vi "svx_Polar_Execute.vi"(0 "Container State":T6, 1 "Polar Plot":refnum<vi>, 2 "Plot Legend":refnum<vi>, 3 "z scale graph":refnum<vi>, 4 "Cursor Info":refnum<vi>, 5 "Facade VI":refnum<vi>, 6 "current state":T1={"Property Name"=[], "Container bounds"={"Width"=550, "Height"=250}, "Scale range"={"Maximum"=1.0, "Increment"=1.0}, "PointIdx"=0, "Marker list"=[], "Color settings"={"Arrow color"=16860, "Magnitude major grid"=13816530, "Magnitude minor grid"=16777216, "Phase grid"=13816530, "Phase scale marker text"=0}, "Magnitude scale name"="Magnitude", "Magnitude scale format string"="%#.2e", "MagnitudeScale:Visible"=TRUE, "MagnitudeScaleLabel:Visible"=TRUE, "PhaseScale:Visible"=TRUE, "Marker:Visible"=TRUE, "Cursor:Visible"=FALSE, "CursorName:Visible"=TRUE, "Autoscale"=TRUE, "Marker color"=16860, "Line color"=16711680, "Cursor color"=16711680, "Magnitude scale marker color"=0, "Plot.Line Style"=0, "Plot.Line Width"=0, "Plot.Point Style"=0, "Cursor.Line Style"=0, "Cursor.Line Width"=0, "Cursor.Point Style"=0, "Cursor.Style"=4, "Marker.Point Style"=2, "Point/fill color"=16711680, "Background color"=16777225, "Cursor name"="", "Cursor Release"=refnum, "Scale Range Change"=refnum, "data size(s)"=[], "Selectors:Visible"=TRUE, "Selector:ring Strings"={"Selector:Custom Strings"=FALSE, "Selector:Row Strings []"=[], "Selector:Column Strings []"=[], "User:Row Strings []"=[], "User:Column Strings []"=[]}, "Lock Cursor Info Position"=FALSE, "CursLoc"={"magnitude"=0.0, "phase"=0.0, "time/rev/RPM"=0.0}, "Plot Area:Position"={"Left"=0, "Top"=0}, "Plot Area:Size"={"Width"=0, "Height"=0}, "Marker.Style"=0, "Indication Arcs"=[], "Arc.Selector"=0, "customized marker"=[], "tree Width"=0, " Parents Tags"=[], "Children Tags"=[], "open?"=[], "index"=[{"row index"=0, "column index"=0}], "Label"="", "custom strings changed"=FALSE, "Owning VI"=refnum, "Legend BG color"=16777225, "Legend font color"=0, "column Width"=203, "attribute"=variant} caption="State", 7 "To Do":T5[](array[typedef]), 8 "Data In":T4) -> (10 "Data Out":T4, 12 "Display State Out":T1={"Property Name"=[], "Container bounds"={"Width"=550, "Height"=250}, "Scale range"={"Maximum"=1.0, "Increment"=1.0}, "PointIdx"=0, "Marker list"=[], "Color settings"={"Arrow color"=16860, "Magnitude major grid"=13816530, "Magnitude minor grid"=16777216, "Phase grid"=13816530, "Phase scale marker text"=0}, "Magnitude scale name"="Magnitude", "Magnitude scale format string"="%#.2e", "MagnitudeScale:Visible"=TRUE, "MagnitudeScaleLabel:Visible"=TRUE, "PhaseScale:Visible"=TRUE, "Marker:Visible"=TRUE, "Cursor:Visible"=FALSE, "CursorName:Visible"=TRUE, "Autoscale"=TRUE, "Marker color"=16860, "Line color"=16711680, "Cursor color"=16711680, "Magnitude scale marker color"=0, "Plot.Line Style"=0, "Plot.Line Width"=0, "Plot.Point Style"=0, "Cursor.Line Style"=0, "Cursor.Line Width"=0, "Cursor.Point Style"=0, "Cursor.Style"=4, "Marker.Point Style"=2, "Point/fill color"=16711680, "Background color"=16777225, "Cursor name"="", "Cursor Release"=refnum, "Scale Range Change"=refnum, "data size(s)"=[], "Selectors:Visible"=TRUE, "Selector:ring Strings"={"Selector:Custom Strings"=FALSE, "Selector:Row Strings []"=[], "Selector:Column Strings []"=[], "User:Row Strings []"=[], "User:Column Strings []"=[]}, "Lock Cursor Info Position"=FALSE, "CursLoc"={"magnitude"=0.0, "phase"=0.0, "time/rev/RPM"=0.0}, "Plot Area:Position"={"Left"=0, "Top"=0}, "Plot Area:Size"={"Width"=0, "Height"=0}, "Marker.Style"=0, "Indication Arcs"=[], "Arc.Selector"=0, "customized marker"=[], "tree Width"=203, " Parents Tags"=[], "Children Tags"=[], "open?"=[], "index"=[{"row index"=0, "column index"=0}], "Label"="", "custom strings changed"=FALSE, "Owning VI"=refnum, "Legend BG color"=16777225, "Legend font color"=0, "column Width"=203, "attribute"=variant} caption="State")   [LabVIEW 2017, in "SVX Polar Plot.xctl"]
uses:
  <vilib>/addons/_XControls/Polar Plot/SVX Polar Plot.xctl
  <vilib>/addons/_XControls/Polar Plot/subVIs/svx_Polar_Plot_Data.ctl
  <vilib>/_xctls/Container State.ctl
  <vilib>/addons/_XControls/Polar Plot/subVIs/svx_Polar_Exe_Tasks.ctl
  <vilib>/addons/_XControls/Polar Plot/subVIs/svx_Polar_Plot_Internal_State.ctl
  <vilib>/addons/_XControls/Polar Plot/subVIs/svx_Polar_Indication_Arcs.ctl
  <vilib>/addons/_XControls/Polar Plot/subVIs/svx_Polar_Customized_Markers.ctl
  <vilib>/Utility/miscctls.llb/LVPointTypeDef.ctl
  <vilib>/Utility/miscctls.llb/LVAnnotationListTypeDef.ctl
  <vilib>/Utility/miscctls.llb/LVBoundsTypeDef.ctl
  <vilib>/_xctls/XControlSupport.lvlib
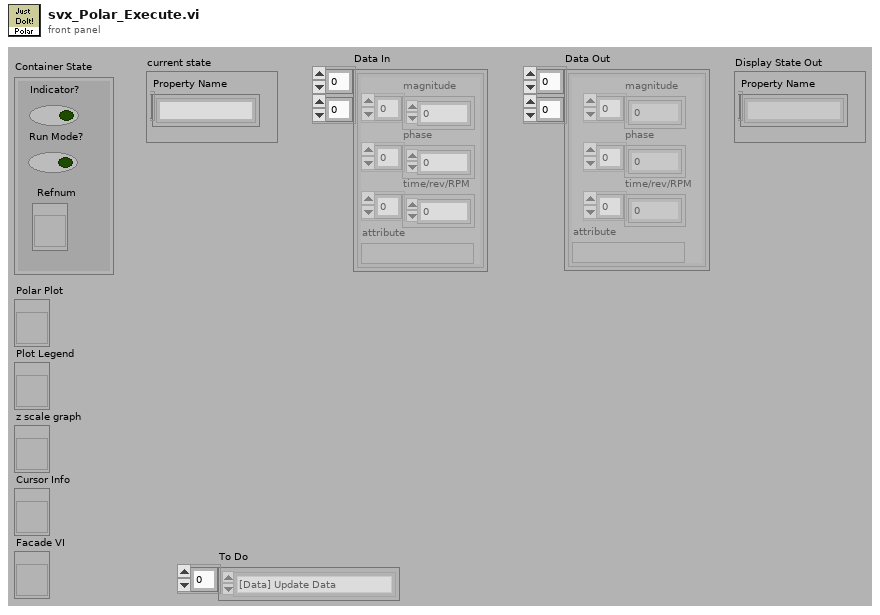
[diagram p1: front panel]
types:
  T1 = typedef "SVX Polar Plot.xctl/svx_Polar_Plot_Internal_State.ctl" = cluster{"Property Name":string[], "Container bounds":cluster{"Width":u32, "Height":u32}, "Scale range":cluster{"Maximum":dbl, "Increment":dbl}, "PointIdx":i32, "Marker list":cluster{"Name":string, "Color":u32, "Style":u8, "Point Style":u8, "Name Visible":bool, "Allow Drag":bool, "Annotation Mode":u32, "Plot":i32, "Index":i32, "Position":cluster{"X":dbl, "Y":dbl}, "X Scale":u32, "Y Scale":u32, "Show Arrow":bool, "Lock Name":bool, "Plot Area":i32, "Label Offset":cluster{"X":dbl, "Y":dbl}}[], "Color settings":cluster{"Arrow color":u32, "Magnitude major grid":u32, "Magnitude minor grid":u32, "Phase grid":u32, "Phase scale marker text":u32}, "Magnitude scale name":string, "Magnitude scale format string":string, "MagnitudeScale:Visible":bool, "MagnitudeScaleLabel:Visible":bool, "PhaseScale:Visible":bool, "Marker:Visible":bool, "Cursor:Visible":bool, "CursorName:Visible":bool, "Autoscale":bool, "Marker color":u32, "Line color":u32, "Cursor color":u32, "Magnitude scale marker color":u32, "Plot.Line Style":i32, "Plot.Line Width":i32, "Plot.Point Style":i32, "Cursor.Line Style":i32, "Cursor.Line Width":i32, "Cursor.Point Style":i32, "Cursor.Style":i32, "Marker.Point Style":i32, "Point/fill color":u32, "Background color":u32, "Cursor name":string, "Cursor Release":refnum<user-event>, "Scale Range Change":refnum<user-event>, "data size(s)":i32[], "Selectors:Visible":bool, "Selector:ring Strings":cluster{"Selector:Custom Strings":bool, "Selector:Row Strings []":string[], "Selector:Column Strings []":string[], "User:Row Strings []":string[], "User:Column Strings []":string[]}, "Lock Cursor Info Position":bool, "CursLoc":cluster{"magnitude":dbl, "phase":dbl, "time/rev/RPM":dbl}, "Plot Area:Position":cluster{"Left":i32, "Top":i32}, "Plot Area:Size":cluster{"Width":u32, "Height":u32}, "Marker.Style":i32, "Indication Arcs":T2, "Arc.Selector":u16, "customized marker":T3, "tree Width":u32, " Parents Tags":string[], "Children Tags":string[], "open?":bool[], "index":cluster{"row index":i32, "column index":i32}[], "Label":string, "custom strings changed":bool, "Owning VI":refnum<vi>, "Legend BG color":u32, "Legend font color":u32, "column Width":u32, "attribute":variant}
  T2 = typedef "SVX Polar Plot.xctl/svx_Polar_Indication_Arcs.ctl" = cluster{"Name":string, "Start radius":dbl, "End radius":dbl, "Line Style":i32, "Line Width":i32, "Border color":u32, "Fill color":u32, "Start angle":i16, "End angle":i16, "Visible":bool}[]
  T3 = typedef "SVX Polar Plot.xctl/svx_Polar_Customized_Markers.ctl" = cluster{"Name":string, "Color":u32, "Style":u8, "Point Style":u8, "Name Visible":bool, "Allow Drag":bool, "Annotation Mode":u32, "Plot":i32, "Index":i32, "Position":cluster{"Magnitude":dbl, "Phase":dbl}, "X Scale":u32, "Y Scale":u32, "Show Arrow":bool, "Lock Name":bool, "Plot Area":i32, "Label Offset":cluster{"Magnitude":dbl, "Phase":dbl}}[]
  T4 = typedef "SVX Polar Plot.xctl/svx_Polar_Plot_Data.ctl" = cluster{"magnitude":dbl[], "phase":dbl[], "time/rev/RPM":dbl[], "attribute":variant}[][]
  T5 = typedef "SVX Polar Plot.xctl/svx_Polar_Exe_Tasks.ctl" = enum16{"[Data] Update Data", "[Scale] Update Polar Scale", "[Scale] Autoscale", "[Legend] Update Legend", "[Cursor] Cursor Release", "[Pane] Change Minimum Size", "[Annt] Upodate Annotation", "[Plot] Appearance", "[Cursor] Visibility", "[Cursor] Appearance", "[Cursor] Index", "[Scale] MagnitudeVisibility", "[Scale] PhaseVisibility", "[Scale] PhaseAppearance", "[Scale] MagnitudeApperance", "[Plot] AcceptanceRegion", "[Scale] RangeChange", "[Marker] Appearance", "[Marker] List", "[Marker] Visibility", "[Legend] Visibility", "[Legend] Color", "[Data] Index", "[Legend] Update String", "[Cursor] Trigger Event", "[Scale] Trigger Event", "[Data] Clear Graph"}
  T6 = typedef "XControlSupport.lvlib/Container State.ctl" = cluster{"Indicator?":bool, "Run Mode?":bool, " Refnum":refnum<vi>}
  T7 = typedef "LVPointTypeDef.ctl" = cluster{"Horizontal":i16, "Vertical":i16}
  T8 = cluster{"Name":string, "Color":u32, "Style":u8, "Point Style":u8, "Name Visible":bool, "Allow Drag":bool, "Annotation Mode":u32, "Plot":i32, "Index":i32, "Position":cluster{"X":dbl, "Y":dbl}, "X Scale":u32, "Y Scale":u32, "Show Arrow":bool, "Lock Name":bool, "Plot Area":i32, "Label Offset":cluster{"X":dbl, "Y":dbl}}[]
  T9 = typedef "LVAnnotationListTypeDef.ctl" = cluster{"Name":string, "Color":u32, "Style":u8, "Point Style":u8, "Name Visible":bool, "Allow Drag":bool, "Annotation Mode":u32, "Plot":i32, "Index":i32, "Position":cluster{"X":dbl, "Y":dbl}, "X Scale":u32, "Y Scale":u32, "Show Arrow":bool, "Lock Name":bool, "Plot Area":i32, "Label Offset":cluster{"X":dbl, "Y":dbl}}[]
  T10 = typedef "LVBoundsTypeDef.ctl" = cluster{"Width":u32, "Height":u32}
  T11 = cluster{"PointIdx":i32, "Position":cluster{"Magnitude":dbl, "Phase":dbl, "Reference":dbl}}
  T12 = cluster{"Selector:Custom Strings":bool, "Selector:Row Strings []":string[], "Selector:Column Strings []":string[], "User:Row Strings []":string[], "User:Column Strings []":string[]}
  T13 = cluster{"magnitude":dbl[], "phase":dbl[], "time/rev/RPM":dbl[], "attribute":variant}
  T14 = cluster{"Arrow color":u32, "Magnitude major grid":u32, "Magnitude minor grid":u32, "Phase grid":u32, "Phase scale marker text":u32}
  T15 = cluster{"Numeric":dbl, "Numeric":dbl, "Numeric":dbl}
  T16 = typedef "LVCursorListTypeDef.ctl" = cluster{"Name":string, "Color":u32, "Style":u8, "Point Style":u8, "Name Visible":bool, "Allow Drag":bool, "Cursor Mode":u32, "Plot":i32, "Index":i32, "Position":cluster{"X":dbl, "Y":dbl}, "X Scale":u32, "Y Scale":u32, "Watch Plots":i32[], "Watch All Plots":bool, "Plot Area":i32, "Label Offset":cluster{"X":dbl, "Y":dbl}}[]
  T17 = cluster{"Name":string, "Color":u32, "Style":u8, "Point Style":u8, "Name Visible":bool, "Allow Drag":bool, "Cursor Mode":u32, "Plot":i32, "Index":i32, "Position":cluster{"X":dbl, "Y":dbl}, "X Scale":u32, "Y Scale":u32, "Watch Plots":i32[], "Watch All Plots":bool, "Plot Area":i32, "Label Offset":cluster{"X":dbl, "Y":dbl}}
  T18 = cluster{"Name":string, "Color":u32, "Style":u8, "Point Style":u8, "Name Visible":bool, "Allow Drag":bool, "Annotation Mode":u32, "Plot":i32, "Index":i32, "Position":cluster{"X":dbl, "Y":dbl}, "X Scale":u32, "Y Scale":u32, "Show Arrow":bool, "Lock Name":bool, "Plot Area":i32, "Label Offset":cluster{"X":dbl, "Y":dbl}}
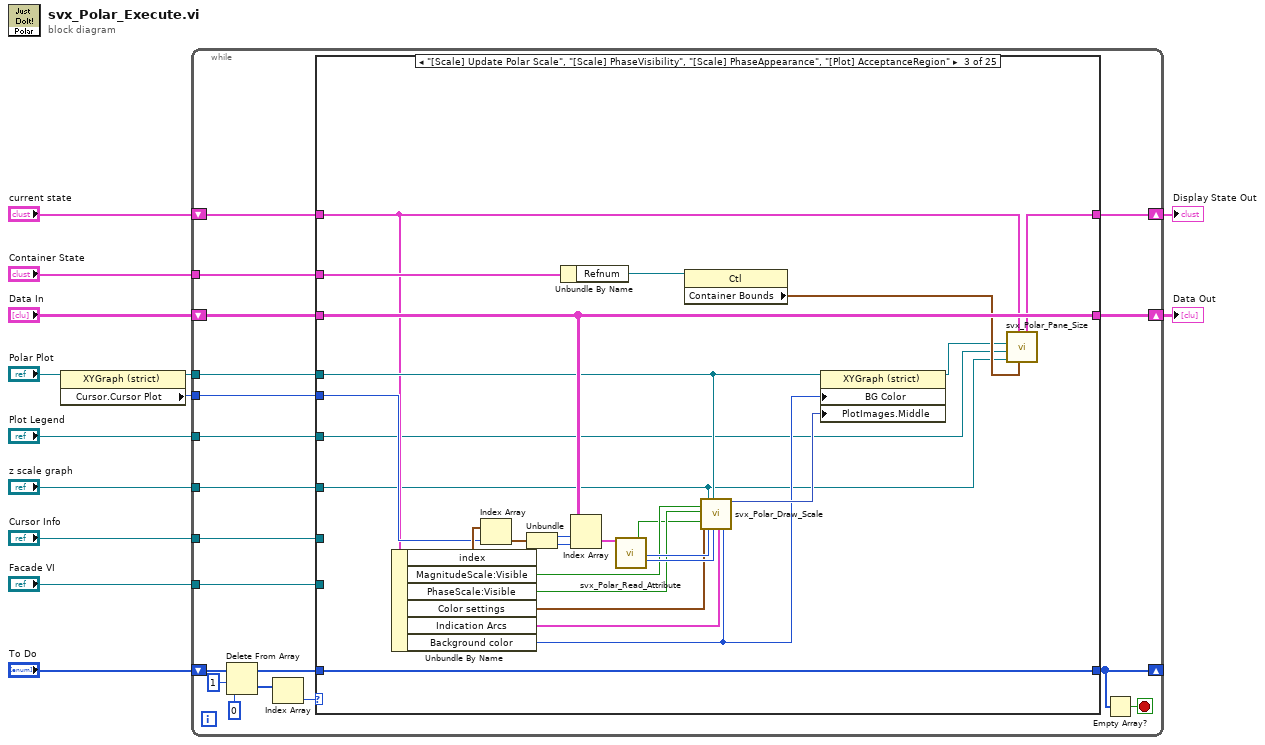
[diagram p0: block diagram]
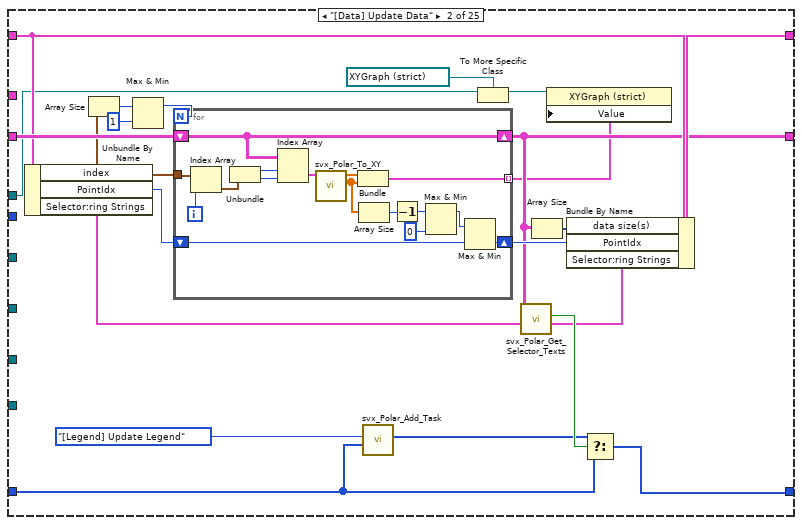
[diagram p3: hidden frame]
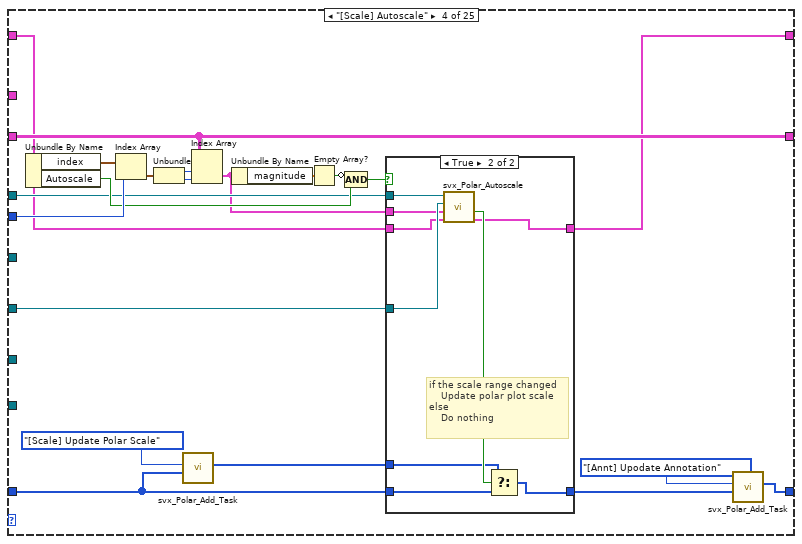
[diagram p4: hidden frame]
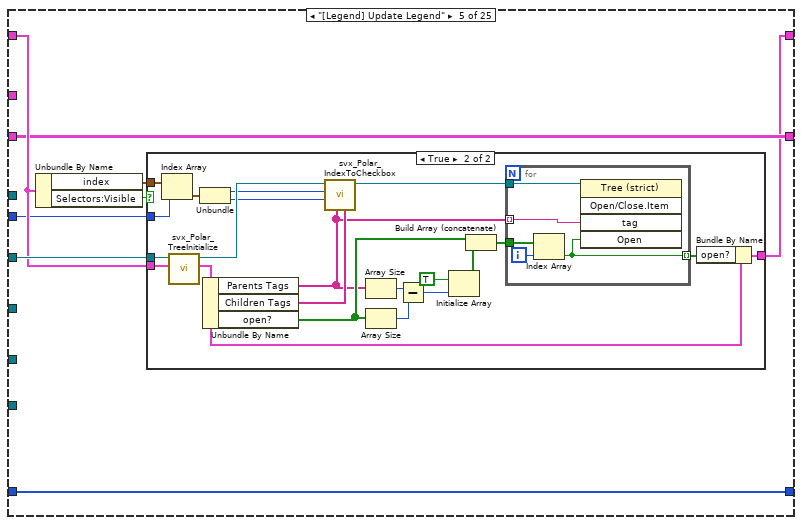
[diagram p6: hidden frame]
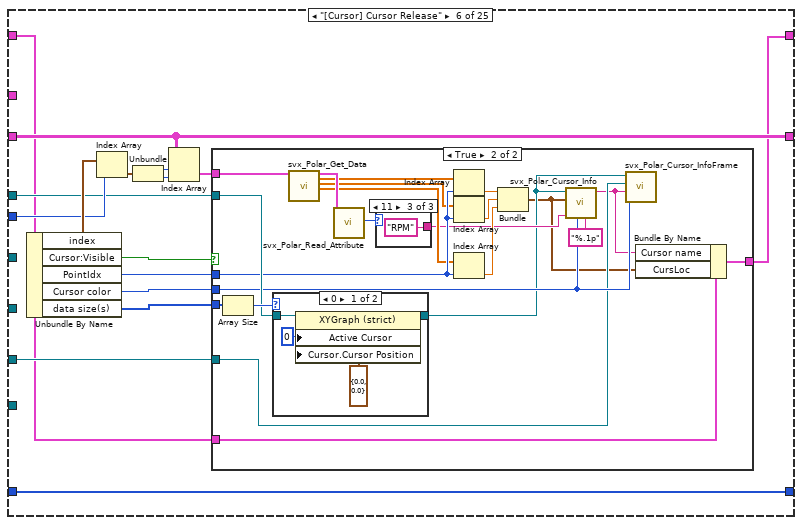
[diagram p8: hidden frame]
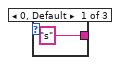
[diagram p10: hidden frame]
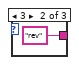
[diagram p11: hidden frame]
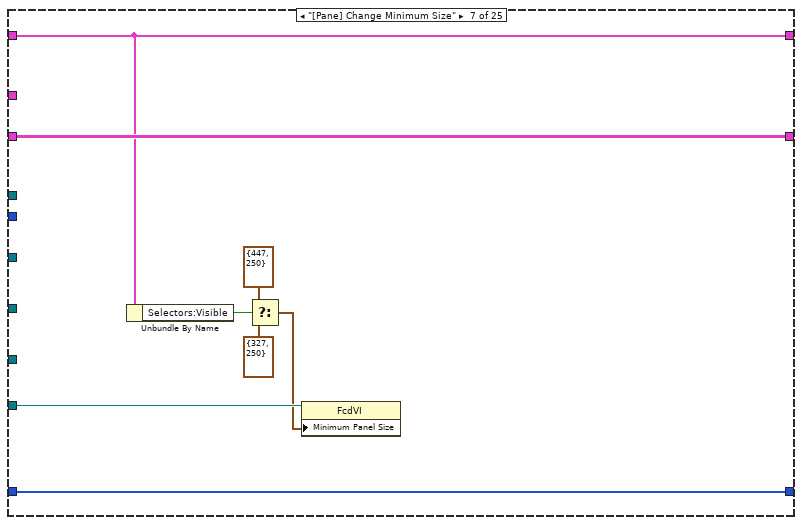
[diagram p13: hidden frame]
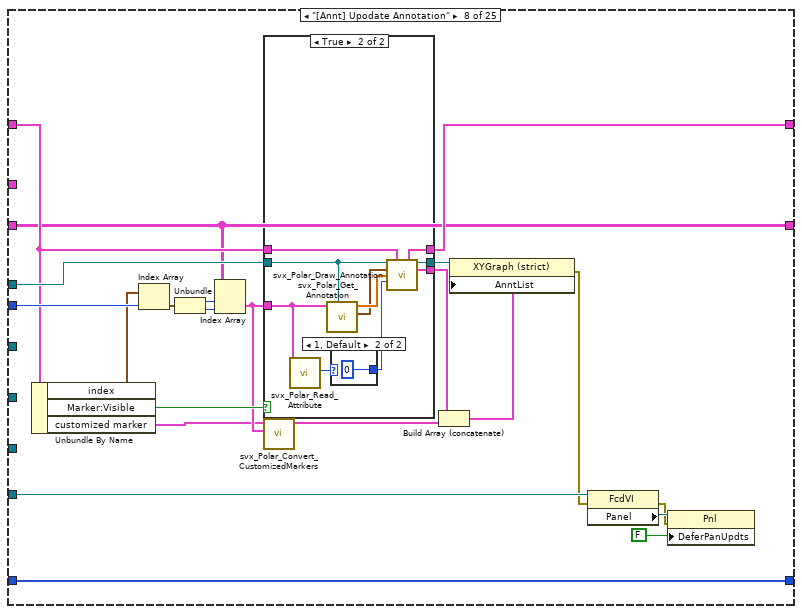
[diagram p14: hidden frame]
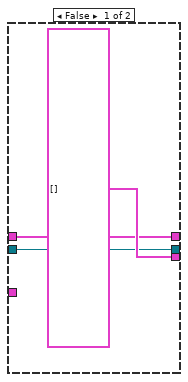
[diagram p15: hidden frame]
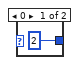
[diagram p16: hidden frame]
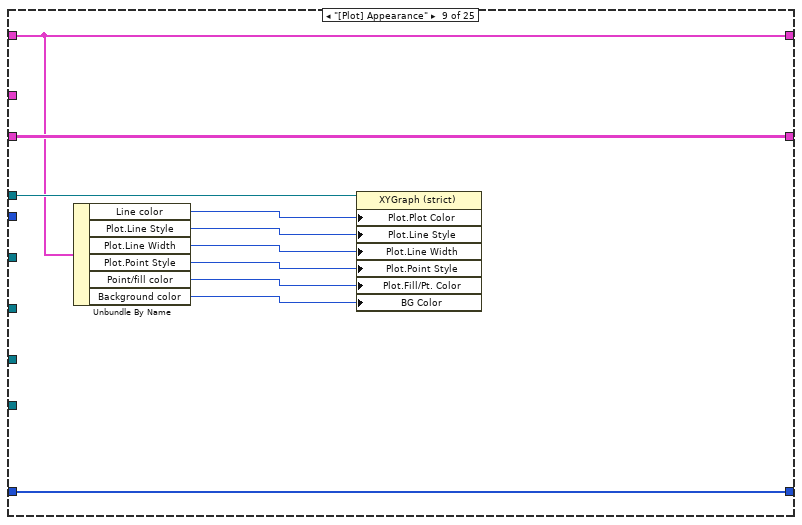
[diagram p17: hidden frame]
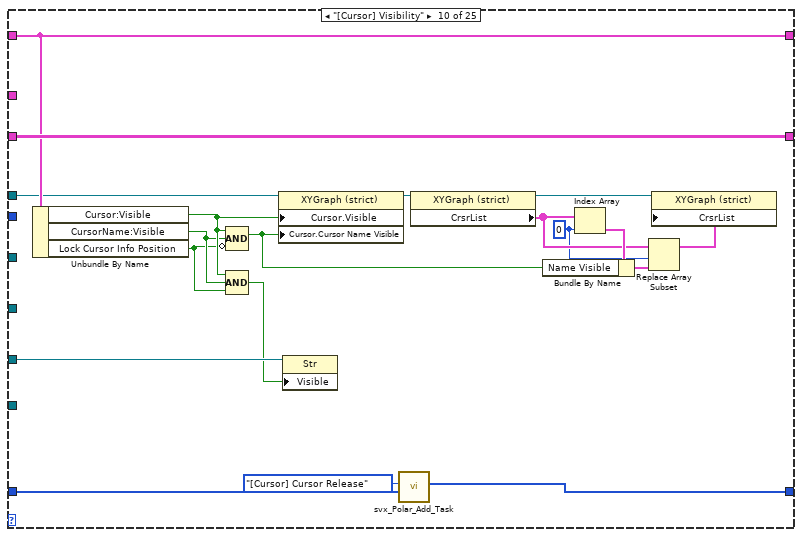
[diagram p18: hidden frame]
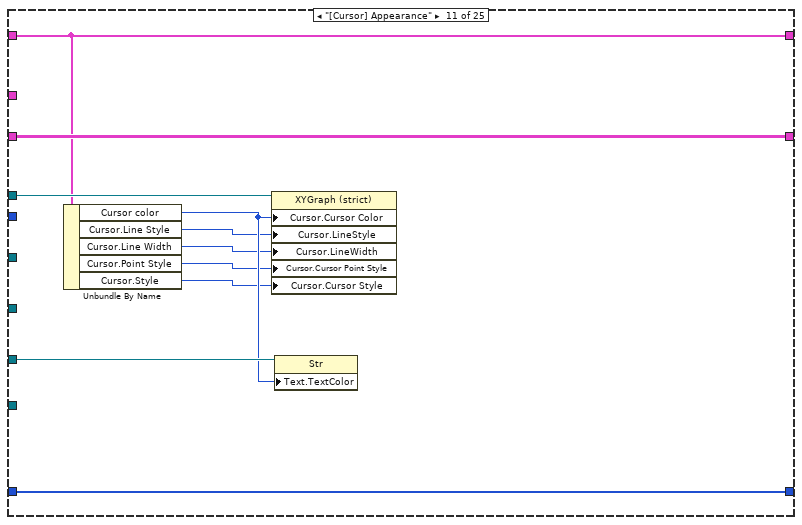
[diagram p19: hidden frame]
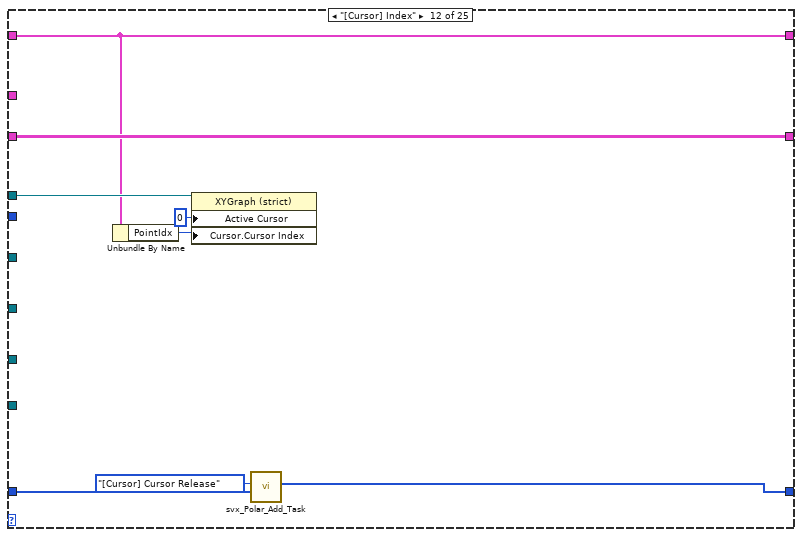
[diagram p20: hidden frame]
diagram:
  n1 = property class="XYGraph (strict)"(reference="Polar Plot") -> (reference out=w10:refnum<vi>, "Cursor.Cursor Plot"=w11:i32)  [unwired: 1 in, 1 out]
  n2 = while {
    shift-right: [w30] -> w6
    shift-left: "current state" -> [w32]
    shift-right: [w14] -> w5
    shift-left: "Data In" -> [w31]
    tunnel: w11 -> [w29]
    tunnel: w10 -> [w28]
    tunnel: "Plot Legend" -> [w27]
    tunnel: "z scale graph" -> [w26]
    tunnel: "Cursor Info" -> [w25]
    shift-right: [w15] -> _
    shift-left: "To Do" -> [w24]
    tunnel: "Facade VI" -> [w17]
    tunnel: "Container State" -> [w16]
    stop <- w19 stop-if-true
    n3 = Delete From Array(array=w24, length=1, index=0) -> (deleted portion=w21:T5[], array with subset deleted=w18:T5[])
    n4 = Index Array(array=w21) -> (element=w20:T5)  [unwired: 1 in]
    n5 = case shown="\"[Scale] Update Polar Scale\", \"[Scale] PhaseVisibility\", \"[Scale] PhaseAppearance\", \"[Plot] AcceptanceRegion\"" w20 {
      tunnel: w32 -> [w35 w55 w78 w107 w138 w169 w217 w236 w265 w283 w294 w301 w307 w329 w348 w363 w375 w392 w439 w447 w457 w469 w478 w484 w491]
      tunnel: w31 -> [w34 w57 w97 w117 w134 w177 w221 w226 w268 w284 w297 w305 w319 w342 w358 w365 w376 w384 w445 w452 w456 w462 w481 w486 _]
      tunnel: [w35 w53 w77 w106 w133 w168 w217 w235 w265 w283 w294 w301 w306 w328 w348 w361 w375 w393 w438 w447 w457 w470 w478 w484 w490] -> w30
      tunnel: w29 -> [_ _ w98 w118 w137 w178 _ w240 _ _ _ _ _ _ _ _ _ w386 _ _ _ _ _ _ _]
      tunnel: w28 -> [_ w43 w85 w110 _ w171 _ w237 w266 w282 w295 w302 w318 w330 w349 w362 w378 w391 w444 _ _ _ _ _ _]
      tunnel: w27 -> [_ _ w75 _ w139 _ _ _ _ _ _ _ w311 w327 _ _ _ _ w443 w446 _ _ _ _ _]
      tunnel: w26 -> [_ _ w74 w109 _ _ _ _ _ _ _ _ w317 w341 w350 _ _ _ w442 _ _ _ _ _ _]
      tunnel: w25 -> [_ _ _ _ _ w170 _ _ _ w278 w293 _ _ _ _ _ _ _ _ _ _ _ _ _ _]
      tunnel: w18 -> [w33 w45 w83 w103 w132 w167 w214 w227 w267 w287 w296 w300 w320 w336 w347 w364 w377 w396 w437 w451 w454 w464 w480 w485 w488]
      tunnel: [w33 w48 w83 w100 w132 w167 w214 w227 w267 w286 w296 w298 w320 w334 w343 w364 w377 w396 w436 w451 w453 w463 w480 w485 w487] -> w15
      tunnel: w17 -> [_ _ _ _ _ _ w216 w231 _ _ _ _ _ _ _ _ _ w383 _ _ _ _ _ _ _]
      tunnel: w16 -> [_ _ w79 _ _ _ _ _ _ _ _ _ w310 w331 _ _ _ _ w441 _ _ _ _ _ _]
      tunnel: [w34 w51 w97 w117 w134 w177 w221 w226 w268 w284 w297 w305 w319 w342 w358 w365 w376 w384 w445 w452 w456 w462 w481 w486 T4 [] ("Data In")] -> w14
      frame Default {
      }
      frame "[Data] Update Data" {
        n6 = Unbundle By Name(w55) -> ("index"=w36:cluster{"row index":i32, "column index":i32}[], "PointIdx"=w56:i32, "Selector:ring Strings"=w50:T12)
        n7 = Array Size(array=w36) -> (size(s)=w38:i32)
        n8 = Max & Min(x=w38, y=1 ("x")) -> (max(x,y)=w39:i32)  [unwired: 1 out]
        n9 = for {
          N: w39 -> [_]
          shift-right: [w73] -> w51
          shift-left: w57 -> [w73]
          tunnel: [w68] -> w40 mode=indexing
          shift-right: [w61] -> w54
          shift-left: w56 -> [w62]
          tunnel: w36 -> [w60]
          i -> [w59]
          n10 = Index Array(array=w60, index=w59) -> (element=w58:cluster{"row index":i32, "column index":i32})
          n11 = Unbundle(w58) -> ("row index"=w72:i32, "column index"=w71:i32)
          n12 = Index Array(array=w73, index (row)=w72, index (col)=w71) -> (element=w70:T13)
          n13 = call <vilib>:"svx_Polar_To_XY.vi"("polar plot"=w70) -> ("y"=w67:dbl[], "x"=w69:dbl[])  [unwired: 7 in, 2 out]
          n14 = Bundle("x"=w69, "y"=w67) -> (w68:cluster{"x":dbl[], "y":dbl[]})  [unwired: 1 in]
          n15 = Array Size(array=w67) -> (size(s)=w65:i32)
          n16 = Decrement(x=w65) -> (x-1=w66:i32)
          n17 = Max & Min(x=w66, y=0) -> (max(x,y)=w63:i32)  [unwired: 1 out]
          n18 = Max & Min(x=w63, y=w62) -> (min(x,y)=w61:i32)  [unwired: 1 out]
        }
        n19 = call <vilib>:"svx_Polar_Add_Task.vi"("task list"=w45, "new task"=svx_Polar_Exe_Tasks."[Legend] Update Legend" ("Tasks")) -> ("task list out"=w44:T5[])  [unwired: 9 in]
        n20 = To More Specific Class(target class=refnum<vi> refnum ("Polar Plot dummy"), reference=w43) -> (specific class reference=w41:refnum<vi>)  [unwired: 1 in, 1 out]
        n21 = call <vilib>:"svx_Polar_Get_Selector_Texts.vi"("Selector:ring Strings"=w50, "polar plot"=w51) -> ("Selector:ring Strings out"=w47:T12, "update legend?"=w49:bool)  [unwired: 7 in, 1 out]
        n22 = Array Size(array=w51) -> (size(s)=w52:i32[])
        n23 = property class="XYGraph (strict)"(reference=w41, "Value"=w40) -> ()  [unwired: 1 in, 2 out]
        n24 = Bundle By Name(cluster=w55, "data size(s)"=w52, "PointIdx"=w54, "Selector:ring Strings"=w47) -> (w53:T1)
        n25 = Select(t=w44, s=w49, f=w45) -> (s? t:f=w48:T5[])
      }
      frame "[Scale] Update Polar Scale", "[Scale] PhaseVisibility", "[Scale] PhaseAppearance", "[Plot] AcceptanceRegion" {
        n26 = Unbundle By Name(w78) -> ("index"=w99:cluster{"row index":i32, "column index":i32}[], "MagnitudeScale:Visible"=w89:bool, "PhaseScale:Visible"=w88:bool, "Color settings"=w86:T14, "Indication Arcs"=w90:T2, "Background color"=w82:u32)
        n27 = Index Array(array=w99, index=w98) -> (element=w96:cluster{"row index":i32, "column index":i32})
        n28 = Unbundle(w96) -> ("row index"=w95:i32, "column index"=w94:i32)
        n29 = Unbundle By Name(w79) -> ("Refnum"=w81:refnum<vi>)
        n30 = Index Array(array=w97, index (row)=w95, index (col)=w94) -> (element=w93:T13)
        n31 = call <vilib>:"svx_Polar_Read_Attribute.vi"("polar plot"=w93) -> ("is OA Polar Plot?"=w87:bool, "shaft rotating direction"=w92:u16, "probe angle [deg]"=w91:u16)  [unwired: 13 in, 3 out]
        n32 = property class="Ctl"(reference=w81) -> ("Container Bounds"=w80:T10)  [unwired: 1 in, 2 out]
        n33 = call <vilib>:"svx_Polar_Draw_Scale.vi"("horizontal line visible"=w89, "thetaScale visible"=w88, "draw rotating direct"=w87, "color settings"=w86, "z scale graph ref in"=w74, "shaft rotating direction"=w92, "Polar Plot ref in"=w85, "probe angle [deg]"=w91, "Indication Arcs"=w90, "Background color"=w82) -> ("new picture"=w84:picture)  [unwired: 9 in]
        n34 = property class="XYGraph (strict)"(reference=w85, "BG Color"=w82, "PlotImages.Middle"=w84) -> (reference out=w76:refnum<vi>)  [unwired: 1 in, 1 out]
        n35 = call <vilib>:"svx_Polar_Pane_Size.vi"("Container bounds"=w80, "Display State In"=w78, "z scale graph Refnum"=w74, "Plot Legend Refnum"=w75, "Polar Plot Refnum in"=w76) -> ("Display State out"=w77:T1)  [unwired: 3 in, 3 out]
      }
      frame "[Scale] Autoscale" {
        n36 = Unbundle By Name(w107) -> ("index"=w119:cluster{"row index":i32, "column index":i32}[], "Autoscale"=w112:bool)
        n37 = Index Array(array=w119, index=w118) -> (element=w120:cluster{"row index":i32, "column index":i32})
        n38 = Unbundle(w120) -> ("row index"=w116:i32, "column index"=w115:i32)
        n39 = call <vilib>:"svx_Polar_Add_Task.vi"("task list"=w103, "new task"=svx_Polar_Exe_Tasks."[Scale] Update Polar Scale" ("element")) -> ("task list out"=w102:T5[])  [unwired: 9 in]
        n40 = Index Array(array=w117, index (row)=w116, index (col)=w115) -> (element=w108:T13)
        n41 = Unbundle By Name(w108) -> ("magnitude"=w113:dbl[])
        n42 = Empty Array?(array=w113) -> (empty?=w114:bool)
        n43 = Compound Arithmetic op=AND(invert w114, w112) -> (w111:bool)
        n44 = case shown="True" w111 {
          tunnel: w110 -> [_ w131]
          tunnel: w109 -> [_ w130]
          tunnel: w108 -> [_ w129]
          tunnel: w107 -> [w121 w128]
          tunnel: w103 -> [w122 w125]
          tunnel: w102 -> [_ w126]
          tunnel: [w122 w124] -> w101
          tunnel: [w121 w123] -> w106
          frame False {
          }
          frame True {
            # "if the scale range changed\n    Update polar plot scale\nelse\n    Do nothing"
            n45 = call <vilib>:"svx_Polar_Autoscale.vi"("State"=w128, "polar plot"=w129, "z scale graph"=w130, "Polar Plot"=w131) -> ("State out"=w123:T1, "redraw scale?"=w127:bool)  [unwired: 4 in, 2 out]
            n46 = Select(t=w126, s=w127, f=w125) -> (s? t:f=w124:T5[])
          }
        }
        n47 = call <vilib>:"svx_Polar_Add_Task.vi"("task list"=w101, "new task"=svx_Polar_Exe_Tasks."[Annt] Upodate Annotation" ("element")) -> ("task list out"=w100:T5[])  [unwired: 9 in]
      }
      frame "[Legend] Update Legend" {
        n48 = Unbundle By Name(w138) -> ("index"=w135:cluster{"row index":i32, "column index":i32}[], "Selectors:Visible"=w136:bool)
        n49 = case shown="True" w136 {
          tunnel: w139 -> [_ w161]
          tunnel: w138 -> [w140 w160]
          tunnel: w135 -> [_ w157]
          tunnel: w137 -> [_ w156]
          tunnel: [w140 w141] -> w133
          frame False {
          }
          frame True {
            n50 = Index Array(array=w157, index=w156) -> (element=w158:cluster{"row index":i32, "column index":i32})
            n51 = call <vilib>:"svx_Polar_TreeInitialize.vi"("Display State In"=w160, "Tree ref in"=w161) -> ("Display State out"=w143:T1, "Tree ref out"=w159:refnum<vi>)  [unwired: 6 in, 2 out]
            n52 = Unbundle(w158) -> ("row index"=w154:i32, "column index"=w155:i32)
            n53 = Unbundle By Name(w143) -> ("Parents Tags"=w146:string[], "Children Tags"=w153:string[], "open?"=w147:bool[])
            n54 = call <vilib>:"svx_Polar_IndexToCheckbox.vi"("All Children Tags"=w153, "All parents Tags"=w146, "ColumnIdx"=w155, "RowIdx"=w154, "Tree ref in"=w159) -> ("Tree ref out"=w144:refnum<vi>)  [unwired: 6 in]
            n55 = Array Size(array=w146) -> (size(s)=w150:i32)
            n56 = Array Size(array=w147) -> (size(s)=w149:i32)
            n57 = Subtract(x=w150, y=w149) -> (x-y=w151:i32)
            n58 = Initialize Array(TRUE, w151) -> (w148:bool[])
            n59 = Build Array (concatenate)(w147, w148) -> (w145:bool[])
            n60 = for {
              tunnel: w144 -> [w166]
              tunnel: w146 -> [w163] mode=indexing
              tunnel: w145 -> [w165]
              tunnel: [w162] -> w142 mode=indexing
              i -> [w164]
              n61 = Index Array(array=w165, index=w164) -> (element=w162:bool)
              n62 = invoke class="Tree (strict)" method="Open/Close.Item"(reference=w166, "tag"=w163, "Open"=w162) -> ()  [unwired: 2 in, 5 out]
            }
            n63 = Bundle By Name(cluster=w143, "open?"=w142) -> (w141:T1)
          }
        }
      }
      frame "[Cursor] Cursor Release" {
        n64 = Unbundle By Name(w169) -> ("index"=w182:cluster{"row index":i32, "column index":i32}[], "Cursor:Visible"=w175:bool, "PointIdx"=w174:i32, "Cursor color"=w173:u32, "data size(s)"=w172:i32[])
        n65 = Index Array(array=w182, index=w178) -> (element=w181:cluster{"row index":i32, "column index":i32})
        n66 = Unbundle(w181) -> ("row index"=w180:i32, "column index"=w179:i32)
        n67 = Index Array(array=w177, index (row)=w180, index (col)=w179) -> (element=w176:T13)
        n68 = case shown="True" w175 {
          tunnel: w176 -> [_ w188]
          tunnel: w174 -> [_ w197]
          tunnel: w173 -> [_ w191]
          tunnel: w172 -> [_ w204]
          tunnel: w171 -> [_ w203]
          tunnel: w170 -> [_ w189]
          tunnel: w169 -> [w183 w187]
          tunnel: [w183 w184] -> w168
          frame False {
          }
          frame True {
            n69 = Array Size(array=w204) -> (size(s)=w205:i32)
            n70 = case shown="0" w205 {
              tunnel: w203 -> [w210 w213]
              tunnel: [w209 w213] -> w190
              frame 0 {
                n71 = property on="Property Node" class="XYGraph (strict)"(reference=w210, "Active Cursor"=u32 0, "Cursor.Cursor Position"=cluster{"Cursor X":dbl, "Cursor Y":dbl} {"Cursor X"=0.0, "Cursor Y"=0.0}) -> (reference out=w209:refnum<vi>)  [unwired: 1 in, 1 out]
              }
              frame 1, Default {
              }
            }
            n72 = call <vilib>:"svx_Polar_Get_Data.vi"("polar plot"=w188) -> ("polar plot out"=w201:T13, "magnitude"=w196:dbl[], "phase"=w195:dbl[], "time/rev/RPM"=w194:dbl[])  [unwired: 13 in, 2 out]
            n73 = call <vilib>:"svx_Polar_Read_Attribute.vi"("polar plot"=w201) -> ("reference label"=w202:u16)  [unwired: 13 in, 5 out]
            n74 = case shown="11" w202 {
              tunnel: ["s" "rev" "RPM"] -> w192
              frame 0, Default {
              }
              frame 3 {
              }
              frame 11 {
              }
            }
            n75 = Index Array(array=w196, index=w197) -> (element=w198:dbl)
            n76 = Index Array(array=w195, index=w197) -> (element=w199:dbl)
            n77 = Index Array(array=w194, index=w197) -> (element=w200:dbl)
            n78 = Bundle("Numeric"=w198, "Numeric"=w199, "Numeric"=w200) -> (w185:T15)  [unwired: 1 in]
            n79 = call <vilib>:"svx_Polar_Cursor_Info.vi"("format string"="%.1p", "cursor color(blue)"=w191, "mark unit"=w192, "CursLoc"=w185, "Polar Plot"=w190) -> ("cursor name"=w186:string)  [unwired: 6 in]
            n80 = call <vilib>:"svx_Polar_Cursor_InfoFrame.vi"("Cursor color"=w191, "format string"=w186, "Cursor Info"=w189, "Polar Plot"=w190) -> ()  [unwired: 8 in]
            n81 = Bundle By Name(cluster=w187, "Cursor name"=w186, "CursLoc"=w185) -> (w184:T1)
          }
        }
      }
      frame "[Pane] Change Minimum Size" {
        n82 = Unbundle By Name(w217) -> ("Selectors:Visible"=w220:bool)
        n83 = Select(t=T7 {"Horizontal"=447, "Vertical"=250} ("Front Panel Window:Minimum Size"), s=w220, f=T7 {"Horizontal"=327, "Vertical"=250} ("Front Panel Window:Minimum Size")) -> (s? t:f=w215:T7)
        n84 = property class="FcdVI"(reference=w216, "Minimum Panel Size"=w215) -> ()  [unwired: 1 in, 2 out]
      }
      frame "[Annt] Upodate Annotation" {
        n85 = Unbundle By Name(w236) -> ("index"=w239:cluster{"row index":i32, "column index":i32}[], "Marker:Visible"=w238:bool, "customized marker"=w224:T3)
        n86 = Index Array(array=w239, index=w240) -> (element=w243:cluster{"row index":i32, "column index":i32})
        n87 = Unbundle(w243) -> ("row index"=w242:i32, "column index"=w241:i32)
        n88 = Index Array(array=w226, index (row)=w242, index (col)=w241) -> (element=w234:T13)
        n89 = case shown="True" w238 {
          tunnel: w234 -> [_ w252]
          tunnel: w237 -> [w244 w251]
          tunnel: w236 -> [w245 w250]
          tunnel: [w245 w249] -> w235
          tunnel: [T8 [] ("AnntList") w248] -> w233
          tunnel: [w244 w247] -> w232
          frame False {
          }
          frame True {
            n90 = call <vilib>:"svx_Polar_Read_Attribute.vi"("polar plot"=w252) -> ("reference label"=w256:u16)  [unwired: 13 in, 5 out]
            n91 = call <vilib>:"svx_Polar_Get_Annotation.vi"("Polar Plot"=w251, "data"=w252) -> ("Array"=w253:cluster{dbl, dbl}[], "marker value"=w254:dbl[])  [unwired: 8 in]
            n92 = case shown="1, Default" w256 {
              tunnel: [i16 2 ("precision (6)") i16 0 ("precision (6)")] -> w255
              frame 0 {
              }
              frame 1, Default {
              }
            }
            n93 = call <vilib>:"svx_Polar_Draw_Annotation.vi"("Polar Plot ref in"=w251, "State in"=w250, "position array"=w253, "Annotation Values"=w254, "precision (6)"=w255) -> ("State out"=w249:T1, "Polar Plot ref out"=w247:refnum<vi>, "AnntList"=w248:T9)  [unwired: 8 in]
          }
        }
        n94 = call <vilib>:"svx_Polar_Convert_CustomizedMarkers.vi"("polar plot"=w234, "customized marker"=w224) -> ("customized annotations"=w222:T9)  [unwired: 9 in]
        n95 = Build Array (concatenate)(w233, w222) -> (w223:T9)
        n96 = property class="XYGraph (strict)"(reference=w232, "AnntList"=w223) -> (error out=w230:errorcluster)  [unwired: 1 in, 1 out]
        n97 = property class="FcdVI"(reference=w231, error in=w230) -> (error out=w225:errorcluster, "Panel"=w229:refnum<vi>)  [unwired: 1 out]
        n98 = property class="Pnl"(reference=w229, error in=w225, "DeferPanUpdts"=FALSE ("Defer Panel Updates")) -> ()  [unwired: 2 out]
      }
      frame "[Plot] Appearance" {
        n99 = Unbundle By Name(w265) -> ("Line color"=w264:u32, "Plot.Line Style"=w263:i32, "Plot.Line Width"=w262:i32, "Plot.Point Style"=w261:i32, "Point/fill color"=w260:u32, "Background color"=w259:u32)
        n100 = property class="XYGraph (strict)"(reference=w266, "Plot.Plot Color"=w264, "Plot.Line Style"=w263, "Plot.Line Width"=w262, "Plot.Point Style"=w261, "Plot.Fill/Pt. Color"=w260, "BG Color"=w259) -> ()  [unwired: 1 in, 2 out]
      }
      frame "[Cursor] Visibility" {
        w274 = 0 ("index")
        n101 = Unbundle By Name(w283) -> ("Cursor:Visible"=w281:bool, "CursorName:Visible"=w280:bool, "Lock Cursor Info Position"=w279:bool)
        n102 = Compound Arithmetic op=AND(w281, w280, invert w279) -> (w271:bool)
        n103 = Compound Arithmetic op=AND(w281, w280, w279) -> (w277:bool)
        n104 = property class="XYGraph (strict)"(reference=w282, "Cursor.Visible"=w281, "Cursor.Cursor Name Visible"=w271) -> (reference out=w270:refnum<vi>)  [unwired: 1 in, 1 out]
        n105 = property class="Str"(reference=w278, "Visible"=w277) -> ()  [unwired: 1 in, 2 out]
        n106 = call <vilib>:"svx_Polar_Add_Task.vi"("task list"=w287, "new task"=svx_Polar_Exe_Tasks."[Cursor] Cursor Release") -> ("task list out"=w286:T5[])  [unwired: 9 in]
        n107 = property class="XYGraph (strict)"(reference=w270) -> (reference out=w272:refnum<vi>, "CrsrList"=w275:T16)  [unwired: 1 in, 1 out]
        n108 = Index Array(array=w275, index=w274) -> (element=w276:T17)
        n109 = Bundle By Name(cluster=w276, "Name Visible"=w271) -> (w273:T17)
        n110 = Replace Array Subset(array=w275, new element=w273, index=w274) -> (w269:T16)
        n111 = property class="XYGraph (strict)"(reference=w272, "CrsrList"=w269) -> ()  [unwired: 1 in, 2 out]
      }
      frame "[Cursor] Appearance" {
        n112 = Unbundle By Name(w294) -> ("Cursor color"=w292:u32, "Cursor.Line Style"=w291:i32, "Cursor.Line Width"=w290:i32, "Cursor.Point Style"=w289:i32, "Cursor.Style"=w288:i32)
        n113 = property class="XYGraph (strict)"(reference=w295, "Cursor.Cursor Color"=w292, "Cursor.LineStyle"=w291, "Cursor.LineWidth"=w290, "Cursor.Cursor Point Style"=w289, "Cursor.Cursor Style"=w288) -> ()  [unwired: 1 in, 2 out]
        n114 = property class="Str"(reference=w293, "Text.TextColor"=w292) -> ()  [unwired: 1 in, 2 out]
      }
      frame "[Cursor] Index" {
        n115 = Unbundle By Name(w301) -> ("PointIdx"=w304:i32)
        n116 = property class="XYGraph (strict)"(reference=w302, "Active Cursor"=u32 0, "Cursor.Cursor Index"=w304) -> ()  [unwired: 1 in, 2 out]
        n117 = call <vilib>:"svx_Polar_Add_Task.vi"("task list"=w300, "new task"=svx_Polar_Exe_Tasks."[Cursor] Cursor Release") -> ("task list out"=w298:T5[])  [unwired: 9 in]
      }
      frame "[Scale] MagnitudeVisibility" {
        n118 = Unbundle By Name(w307) -> ("MagnitudeScale:Visible"=w314:bool, "MagnitudeScaleLabel:Visible"=w315:bool)
        n119 = Unbundle By Name(w310) -> ("Refnum"=w309:refnum<vi>)
        n120 = property class="XYGraph (strict)"(reference=w317, "Visible"=w314, "YScale.NameLbl.Visible"=w315) -> (reference out=w316:refnum<vi>)  [unwired: 1 in, 1 out]
        n121 = property class="Ctl"(reference=w309) -> ("Container Bounds"=w308:T10)  [unwired: 1 in, 2 out]
        n122 = case shown="False" w314 {
          tunnel: w318 -> [w322 w325]
          tunnel: w316 -> [w321 w323]
          tunnel: [w322 w324] -> w313
          tunnel: [w321 w323] -> w312
          frame False {
          }
          frame True {
            n123 = call <vilib>:"svx_Polar_Align_Plot_Area.vi"("z scale graph ref in"=w323, "Polar Plot ref in"=w325) -> ("Polar Plot ref out"=w324:refnum<vi>)  [unwired: 8 in, 1 out]
          }
        }
        n124 = call <vilib>:"svx_Polar_Pane_Size.vi"("Container bounds"=w308, "Display State In"=w307, "z scale graph Refnum"=w312, "Plot Legend Refnum"=w311, "Polar Plot Refnum in"=w313) -> ("Display State out"=w306:T1)  [unwired: 3 in, 3 out]
      }
      frame "[Scale] MagnitudeApperance" {
        n125 = Unbundle By Name(w329) -> ("Color settings.Magnitude major grid"=w340:u32, "Magnitude scale marker color"=w339:u32, "Magnitude scale name"=w338:string, "Magnitude scale format string"=w337:string)
        n126 = Unbundle By Name(w331) -> ("Refnum"=w333:refnum<vi>)
        n127 = property class="Ctl"(reference=w333) -> ("Container Bounds"=w332:T10)  [unwired: 1 in, 2 out]
        n128 = property class="XYGraph (strict)"(reference=w341, "YScale.MinorTickColor"=w340, "YScale.TickColor"=w340, "YScale.Text Color"=w339, "YScale.NameLbl.Text"=w338, "YScale.FormatString"=w337) -> (reference out=w326:refnum<vi>)  [unwired: 1 in, 1 out]
        n129 = call <vilib>:"svx_Polar_Add_Task.vi"("task list"=w336, "new task"=svx_Polar_Exe_Tasks."[Scale] Update Polar Scale") -> ("task list out"=w334:T5[])  [unwired: 9 in]
        n130 = call <vilib>:"svx_Polar_Pane_Size.vi"("Container bounds"=w332, "Display State In"=w329, "z scale graph Refnum"=w326, "Plot Legend Refnum"=w327, "Polar Plot Refnum in"=w330) -> ("Display State out"=w328:T1)  [unwired: 3 in, 3 out]
      }
      frame "[Scale] RangeChange" {
        n131 = Unbundle By Name(w348) -> ("Scale range.Maximum"=w355:dbl)
        n132 = Negate(x=w355) -> (-x=w351:dbl)
        n133 = call <vilib>:"svx_Polar_Add_Task.vi"("task list"=w347, "new task"=svx_Polar_Exe_Tasks."[Scale] Update Polar Scale") -> ("task list out"=w345:T5[])  [unwired: 9 in]
        n134 = property on="Property Node" class="XYGraph (strict)"(reference=w349, "XScale.Maximum"=w355, "XScale.Minimum"=w351, "YScale.Maximum"=w355, "YScale.Minimum"=w351) -> (reference out=w356:refnum<vi>, error out=w354:errorcluster)  [unwired: 1 in]
        n135 = call <vilib>:"svx_Polar_Add_Task.vi"("task list"=w345, "new task"=svx_Polar_Exe_Tasks."[Annt] Upodate Annotation") -> ("task list out"=w343:T5[])  [unwired: 9 in]
        n136 = property on="Property Node" class="XYGraph (strict)"(reference=w350, error in=w354, "YScale.Flipped"=FALSE ("Y Scale.Flipped"), "YScale.Maximum"=w355, "YScale.Minimum"=0.0 ("Minimum")) -> (reference out=w357:refnum<vi>)  [unwired: 1 out]
        n137 = call <vilib>:"svx_Polar_Align_Plot_Area.vi"("z scale graph ref in"=w357, "Polar Plot ref in"=w356) -> ()  [unwired: 8 in, 2 out]
      }
      frame "[Marker] Appearance" {
        n138 = Unbundle By Name(w363) -> ("Marker color"=w369:u32, "Marker.Point Style"=w360:i32, "Marker.Style"=w359:i32)
        n139 = property class="XYGraph (strict)"(reference=w362) -> (reference out=w366:refnum<vi>, "AnntList"=w367:T9)  [unwired: 1 in, 1 out]
        n140 = for {
          tunnel: w367 -> [w374] mode=indexing
          tunnel: w369 -> [w373]
          tunnel: [w372] -> w368 mode=indexing
          tunnel: w360 -> [w371]
          tunnel: w359 -> [w370]
          n141 = Bundle By Name(cluster=w374, "Color"=w373, "Point Style"=w371, "Style"=w370) -> (w372:T18)
        }
        n142 = Bundle By Name(cluster=w363, "Marker list"=w368) -> (w361:T1)
        n143 = property class="XYGraph (strict)"(reference=w366, "AnntList"=w368) -> ()  [unwired: 1 in, 2 out]
      }
      frame "[Marker] List" {
        n144 = Unbundle By Name(w375) -> ("Marker list"=w379:T8)
        n145 = property on="Property Node" class="XYGraph (strict)"(reference=w378, "AnntList"=w379) -> (reference out=w380:refnum<vi>)  [unwired: 1 in, 1 out]
        n146 = property on="Property Node" class="XYGraph (strict)"(reference=w380) -> (reference out=w381:refnum<vi>, "AnntList"=w382:T9)  [unwired: 1 in, 1 out]
        n147 = property on="Property Node" class="XYGraph (strict)"(reference=w381, "AnntList"=w382) -> ()  [unwired: 1 in, 2 out]
      }
      frame "[Marker] Visibility" {
        n148 = Unbundle By Name(w392) -> ("Marker:Visible"=w394:bool, "customized marker"=w395:T3, "index"=w387:cluster{"row index":i32, "column index":i32}[])
        n149 = Index Array(array=w387, index=w386) -> (element=w390:cluster{"row index":i32, "column index":i32})
        n150 = Unbundle(w390) -> ("row index"=w389:i32, "column index"=w388:i32)
        n151 = Index Array(array=w384, index (row)=w389, index (col)=w388) -> (element=w385:T13)
        n152 = case shown="True" w394 {
          selector: w394 -> [w406 _]
          tunnel: w392 -> [w407 w419]
          tunnel: w391 -> [w399 w425]
          tunnel: w385 -> [w400 w415]
          tunnel: [w405 w420] -> w393
          tunnel: w395 -> [w398 w409]
          tunnel: w383 -> [_ w413]
          frame False {
            n153 = call <vilib>:"svx_Polar_Convert_CustomizedMarkers.vi"("polar plot"=w400, "customized marker"=w398) -> ("customized annotations"=w397:T9)  [unwired: 9 in]
            n154 = property class="XYGraph (strict)"(reference=w399, "AnntList"=w397) -> (reference out=w401:refnum<vi>)  [unwired: 1 in, 1 out]
            n155 = property class="XYGraph (strict)"(reference=w401) -> (reference out=w403:refnum<vi>, "AnntList"=w402:T9)  [unwired: 1 in, 1 out]
            n156 = Bundle By Name(cluster=w407, "Marker:Visible"=w406, "Marker list"=T9 [] ("Annotation List")) -> (w405:T1)
            n157 = property class="XYGraph (strict)"(reference=w403, "AnntList"=w402) -> ()  [unwired: 1 in, 2 out]
          }
          frame True {
            # "Do NOT remove this Read/Write operations.\nIt's not redundant. It is used to solve a update problem."
            n158 = call <vilib>:"svx_Polar_Read_Attribute.vi"("polar plot"=w415) -> ("reference label"=w418:u16)  [unwired: 13 in, 5 out]
            n159 = call <vilib>:"svx_Polar_Get_Annotation.vi"("Polar Plot"=w425, "data"=w415) -> ("Array"=w426:cluster{dbl, dbl}[], "marker value"=w427:dbl[])  [unwired: 8 in]
            n160 = case shown="1, Default" w418 {
              tunnel: [i16 2 ("precision (6)") i16 0 ("precision (6)")] -> w428
              frame 0 {
              }
              frame 1, Default {
              }
            }
            n161 = call <vilib>:"svx_Polar_Draw_Annotation.vi"("Polar Plot ref in"=w425, "State in"=w419, "position array"=w426, "Annotation Values"=w427, "precision (6)"=w428) -> ("State out"=w422:T1, "Polar Plot ref out"=w414:refnum<vi>, "AnntList"=w416:T9)  [unwired: 8 in]
            n162 = call <vilib>:"svx_Polar_Convert_CustomizedMarkers.vi"("polar plot"=w415, "customized marker"=w409) -> ("customized annotations"=w408:T9)  [unwired: 9 in]
            n163 = Build Array (concatenate)(w416, w408) -> (w417:T9)
            n164 = property class="XYGraph (strict)"(reference=w414, "AnntList"=w417) -> (reference out=w424:refnum<vi>)  [unwired: 1 in, 1 out]
            n165 = property class="XYGraph (strict)"(reference=w424) -> (reference out=w423:refnum<vi>, "AnntList"=w421:T9)  [unwired: 1 in, 1 out]
            n166 = property class="XYGraph (strict)"(reference=w423, "AnntList"=w421) -> (error out=w412:errorcluster)  [unwired: 1 in, 1 out]
            n167 = property class="FcdVI"(reference=w413, error in=w412) -> ("Panel"=w411:refnum<vi>)  [unwired: 2 out]
            n168 = Bundle By Name(cluster=w422, "Marker list"=w416) -> (w420:T1)
            n169 = property class="Pnl"(reference=w411, "DeferPanUpdts"=FALSE ("Defer Panel Updates")) -> ()  [unwired: 1 in, 2 out]
          }
        }
      }
      frame "[Legend] Visibility" {
        n170 = Unbundle By Name(w441) -> ("Refnum"=w440:refnum<vi>)
        n171 = Unbundle By Name(w439) -> ("Container bounds.Width"=w433:u32, "Container bounds.Height"=w432:u32)
        n172 = call <vilib>:"svx_Polar_Add_Task.vi"("task list"=w437, "new task"=svx_Polar_Exe_Tasks."[Pane] Change Minimum Size") -> ("task list out"=w436:T5[])  [unwired: 9 in]
        n173 = Bundle By Name(cluster=T10 {"Width"=0, "Height"=0} ("Previouse Container bounds"), "Width"=w433, "Height"=w432) -> (w431:T10)
        n174 = call <vilib>:"svx_Polar_Legend_Visible.vi"("Previous Container bounds"=w431, "Display State In"=w439, "z scale graph Refnum"=w442, "Plot Legend Refnum"=w443, "Polar Plot Refnum in"=w444, "Container Refnum"=w440) -> ("Display State out"=w438:T1)  [unwired: 1 in, 4 out]
      }
      frame "[Legend] Color" {
        w448 = -2 ("Active Cell:Active Column Number")
        n175 = Unbundle By Name(w447) -> ("Legend BG color"=w449:u32, "Legend font color"=w450:u32)
        n176 = property class="Tree (strict)"(reference=w446, "ActiveColNum"=w448, "Active Item Row Number"=w448, "CellBG"=w449, "CellFontColor"=w450) -> ()  [unwired: 1 in, 2 out]
      }
      frame "[Data] Index" {
        w455 = T5[] [enum."[Data] Update Data", enum."[Scale] Autoscale", enum."[Cursor] Cursor Release", enum."[Legend] Update Legend"] items=["[Data] Update Data", "[Scale] Update Polar Scale", "[Scale] Autoscale", "[Legend] Update Legend", "[Cursor] Cursor Release", "[Pane] Change Minimum Size", "[Annt] Upodate Annotation", "[Plot] Appearance", "[Cursor] Visibility", "[Cursor] Appearance", "[Cursor] Index", "[Scale] MagnitudeVisibility", "[Scale] PhaseVisibility", "[Scale] PhaseAppearance", "[Scale] MagnitudeApperance", "[Plot] AcceptanceRegion", "[Scale] RangeChange", "[Marker] Appearance", "[Marker] List", "[Marker] Visibility", "[Legend] Visibility", "[Legend] Color", "[Data] Index", "[Legend] Update String", "[Cursor] Trigger Event", "[Scale] Trigger Event", "[Data] Clear Graph"] ("To Do")
        n177 = for {
          tunnel: w455 -> [w459] mode=indexing
          shift-right: [w458] -> w453
          shift-left: w454 -> [w460]
          n178 = call <vilib>:"svx_Polar_Add_Task.vi"("task list"=w460, "new task"=w459) -> ("task list out"=w458:T5[])  [unwired: 9 in]
        }
      }
      frame "[Legend] Update String" {
        n179 = Unbundle By Name(w469) -> ("Selector:ring Strings"=w468:T12)
        n180 = call <vilib>:"svx_Polar_Get_Selector_Texts.vi"("Selector:ring Strings"=w468, "polar plot"=w462) -> ("Selector:ring Strings out"=w471:T12, "update legend?"=w466:bool)  [unwired: 7 in, 1 out]
        n181 = call <vilib>:"svx_Polar_Add_Task.vi"("task list"=w464, "new task"=svx_Polar_Exe_Tasks."[Legend] Update Legend") -> ("task list out"=w465:T5[])  [unwired: 9 in]
        n182 = Array Size(array=w462) -> (size(s)=w461:i32[])
        n183 = Bundle By Name(cluster=w469, "data size(s)"=w461, "Selector:ring Strings"=w471) -> (w470:T1)
        n184 = Select(t=w465, s=w466, f=w464) -> (s? t:f=w463:T5[])
      }
      frame "[Cursor] Trigger Event" {
        n185 = Unbundle By Name(w478) -> ("Cursor Release"=w475:refnum<user-event>, "PointIdx"=w477:i32, "CursLoc.magnitude"=w474:dbl, "CursLoc.phase"=w473:dbl, "CursLoc.time/rev/RPM"=w472:dbl)
        n186 = Bundle By Name(cluster=T11 {"PointIdx"=0, "Position"={"Magnitude"=0.0, "Phase"=0.0, "Reference"=0.0}} ("event data"), "PointIdx"=w477, "Position.Magnitude"=w474, "Position.Phase"=w473, "Position.Reference"=w472) -> (w476:T11)
        n187 = Generate User Event(user event=w475, event data cluster=w476) -> ()  [unwired: 2 in, 2 out]
      }
      frame "[Scale] Trigger Event" {
        n188 = Unbundle By Name(w484) -> ("Scale Range Change"=w483:refnum<user-event>, "Scale range.Maximum"=w482:dbl)
        n189 = Generate User Event(user event=w483, event data cluster=w482) -> ()  [unwired: 2 in, 2 out]
      }
      frame "[Data] Clear Graph" {
        w489 = T5[] [enum."[Data] Update Data", enum."[Scale] Update Polar Scale", enum."[Cursor] Cursor Release", enum."[Annt] Upodate Annotation", enum."[Legend] Update Legend"] items=["[Data] Update Data", "[Scale] Update Polar Scale", "[Scale] Autoscale", "[Legend] Update Legend", "[Cursor] Cursor Release", "[Pane] Change Minimum Size", "[Annt] Upodate Annotation", "[Plot] Appearance", "[Cursor] Visibility", "[Cursor] Appearance", "[Cursor] Index", "[Scale] MagnitudeVisibility", "[Scale] PhaseVisibility", "[Scale] PhaseAppearance", "[Scale] MagnitudeApperance", "[Plot] AcceptanceRegion", "[Scale] RangeChange", "[Marker] Appearance", "[Marker] List", "[Marker] Visibility", "[Legend] Visibility", "[Legend] Color", "[Data] Index", "[Legend] Update String", "[Cursor] Trigger Event", "[Scale] Trigger Event", "[Data] Clear Graph"] ("To Do")
        w497 = string[] [] ("Selector:Row Strings []")
        n190 = Unbundle By Name(w491) -> ("Selector:ring Strings"=w494:T12)
        n191 = Bundle By Name(cluster=w494, "Selector:Row Strings []"=w497, "Selector:Column Strings []"=w497) -> (w495:T12)
        n192 = Bundle By Name(cluster=w491, "PointIdx"=0, "data size(s)"=i32[] [], "Selector:ring Strings"=w495, "customized marker"=T3 []) -> (w490:T1)
        n193 = for {
          tunnel: w489 -> [w499] mode=indexing
          shift-right: [w500] -> w487
          shift-left: w488 -> [w501]
          n194 = call <vilib>:"svx_Polar_Add_Task.vi"("task list"=w501, "new task"=w499) -> ("task list out"=w500:T5[])  [unwired: 9 in]
        }
      }
    }
    n195 = Empty Array?(array=w15) -> (empty?=w19:bool)
  }
  "Display State Out" <- w6
  "Data Out" <- w5
